vi "Make Bias.vi"(8 "error in (no error)":errorcluster, 11 "Setup File in":refnum<class "Setup File.lvclass">) -> (0 "error out":errorcluster, 3 "Setup File out":refnum<class "Setup File.lvclass">)   [LabVIEW 2018, in "Setup File.lvclass"]
doc: "Este VI cria um arquivo texto com a configuração para aquisição de imagens de bias: tempo de exposição igual a zero, shutter constantemente fechado, e pre-amplificação 1."
uses:
  Setup File.lvclass
  Setup File.lvclass/Setup File.ctl
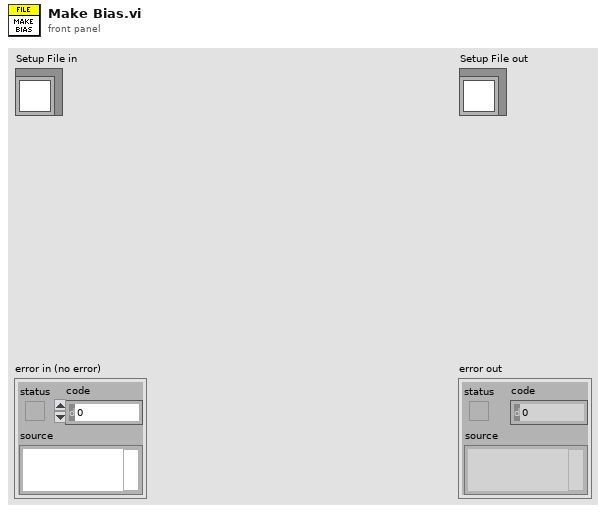
[diagram p1: front panel]
types:
  T1 = enum16{"open", "replace", "create", "open or create", "replace or create", "replace or create with confirmation"}
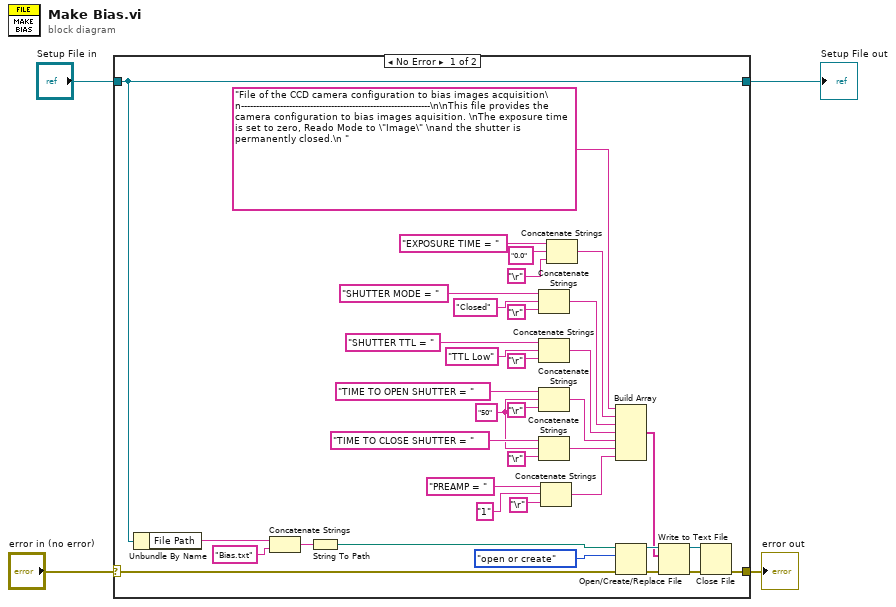
[diagram p0: block diagram]
diagram:
  n1 = case shown="No Error" "error in (no error)" {
    selector: "error in (no error)" -> [w41 w43]
    tunnel: [w38 w43] -> w3
    tunnel: [w35 w42] -> w1
    tunnel: "Setup File in" -> [w35 w42]
    frame No Error {
      w17 = "50"
      n2 = Unbundle By Name(w35) -> ("File Path"=w34:string)
      n3 = Concatenate Strings(w34, "Bias.txt") -> (w33:string)
      n4 = String To Path(string=w33) -> (path=w32:path)
      n5 = Concatenate Strings("SHUTTER MODE = ", "Closed", "\r") -> (w24:string)
      n6 = Concatenate Strings("SHUTTER TTL = ", "TTL Low", "\r") -> (w23:string)
      n7 = Concatenate Strings("TIME TO OPEN SHUTTER = ", w17, "\r") -> (w22:string)
      n8 = Concatenate Strings("TIME TO CLOSE SHUTTER = ", w17, "\r") -> (w8:string)
      n9 = Concatenate Strings("PREAMP = ", "1", "\r") -> (w7:string)
      n10 = Concatenate Strings("EXPOSURE TIME = ", "0.0", "\r") -> (w25:string)
      n11 = Build Array("File of the CCD camera configuration to bias images acquisition\n---------------------------------------------------------------\n\nThis file provides the camera configuration to bias images aquisition. \nThe exposure time is set to zero, Reado Mode to \"Image\" \nand the shutter is permanently closed.\n " ("string"), w25, w24, w23, w22, w8, w7) -> (w21:string[])
      n12 = Open/Create/Replace File(file path (use dialog)=w32, error in=w41, operation (0:open)=T1."open or create") -> (refnum out=w37:refnum<file>, error out=w40:errorcluster)  [unwired: 3 in, 1 out]
      n13 = Write to Text File(file (use dialog)=w37, text=w21, error in=w40) -> (refnum out=w36:refnum<file>, error out=w39:errorcluster)  [unwired: 1 in, 1 out]
      n14 = Close File(refnum=w36, error in=w39) -> (error out=w38:errorcluster)  [unwired: 1 out]
    }
    frame Error {
    }
  }
  "error out" <- w3
  "Setup File out" <- w1
